vi "Controller Monitoring Loop.vi"(7 "Sync Objects":T1, 8 "error in (no error)":errorcluster, 11 "FOFB Configuration":T4={"FOFB Parameters"={"Network"={"FOFB Controller IP"="", "LNLS Control Network IP"="", "LNLS Control Network Power Supplies TCP Port"=0, "LNLS Control Network FOFB Configuration TCP Port"=0, "LNLS Control Network BPMs TCP Port"=0, "Data Server TCP Port"=0, "Monitoring Data TCP Port"=0, "Configuration GUI TCP Port"=0, "Storage Data TCP Port"=0, "Fast Command TCP Port"=0, "TCP Listening Timeout"=0, "Request Setpoints Rate"=0}, "Fast Acquisition"={"Acquisition Period"=0, "Data Buffer Size"=0, "Monitoring Period"=0}, "Response Matrix Measurement"={"Step Amplitude"=0.0, "Time Between Steps"=0, "Step Duration"=0, "Number of Averages"=0}, "Correction Algorithm"={"Correction Period"=0, "Reference Orbit Path"=path "", "Response Matrix Path"=path "", "Correction Matrix Path"=path "", "PID Horizontal Gain"=0.0, "PID Vertical Gain"=0.0, "PID Horizontal Integral Time"=0.0, "PID Vertical Integral Time"=0.0, "PID Horizontal Derivative Time"=0.0, "PID Vertical Derivative Time"=0.0, "Beam Current FOFB Threshold"=0.0, "Decouple H-V"=FALSE, "Use Additional BPM LPF"=FALSE, "BPM LPF Cutoff"=0.0}, "Acquisition Network"=[], "Actuation Network"=[]}, "Number of Acquisition Chassis"=0, "Number of Actuation Chassis"=0, "Number of BPM Readings"=0, "BPM Reading Names"=[], "Selected BPM Readings"=[0, 1, 2, 3, 4, 5, 6, 7, 8, 9, 10, 11, 12, 13, 14, 15, 16, 17, 18, 19, 20, 21, 22, 23, 24, 25, 26, 27, 28, 29, 30, 31, 32, 33, 34, 35, 36, 37, 38, 39, 40, 41, 42, 43, 44, 45, 46, 47, 48, 49], "Number of Correctors"=0, "Corrector Names"=[], "Selected Correctors"=[0, 1, 2, 3, 4, 5, 6, 7, 8, 9, 10, 11, 12, 13, 14, 15, 16, 17, 18, 19, 20, 21, 22, 23, 24, 25, 26, 27, 28, 29, 30, 31, 32, 33, 34, 35, 36, 37, 38, 39, 40, 41, 42, 43, 44, 45, 46, 47, 48, 49], "Reference Orbit"=[], "Response Matrix"=[], "Correction Matrix"=[], "Acquisition Chassis Names"=[], "Actuation Chassis Names"=[], "Acquisition Variables"=[], "Actuation Variables"=[], "PS Matrix Mapping"=[], "Inverse PS Matrix Mapping"=[], "BPM Matrix Mapping"=[], "Inverse BPM Matrix Mapping"=[], "Response Matrix Beam Energy (MeV)"=0.0, "PID Parameters"=[], "BPM Planes"=[], "Corrector Planes"=[], "RMM Step Factor"=[]}) -> (0 "error out":errorcluster)   [LabVIEW 2011, in "Controller VIs.lvlib"]
uses:
  Controller VIs.lvlib
  Types Definitions/Type FOFB Configuration.ctl
  Types Definitions/Type FOFB Parameters.ctl
  Types Definitions/Type Network Configuration.ctl
  Types Definitions/Type FA Configuration.ctl
  Types Definitions/Type Response Matrix Measurement Configuration.ctl
  Types Definitions/Type Correction Algorithm Configuration.ctl
  Types Definitions/Type Acquisition Network Configuration.ctl
  Types Definitions/Type Actuation Network Configuration.ctl
  Types Definitions/Type PID Parameters.ctl
  Types Definitions/Type Synchronization Objects.ctl
  Types Definitions/Type Blocking Synchronization Objects.ctl
  Types Definitions/Type Monitoring Data.ctl
  Types Definitions/Type Operation Mode State.ctl
  Types Definitions/Type Diagnostics Data.ctl
  Types Definitions/Type CPU Loads Array.ctl
  Types Definitions/Type CPU Loads.ctl
  Types Definitions/Type Non-blocking Synchronization Objects.ctl
  Types Definitions/Type FOFB Variables.ctl
  Types Definitions/Type Actuation State.ctl
  Types Definitions/Type TCP State.ctl
  <vilib>/Platform/TimedLoop/XDataNode/timing_clust.ctl
  <vilib>/Platform/TimedLoop/XDataNode/nitl_modes.ctl
  <vilib>/Platform/TimedLoop/XDataNode/wakeup.ctl
  Controller Global Variables/Controller Actuation State.vi
  Controller Global Variables/LNLS Control FOFB Configuration Out.vi
  Controller Global Variables/Monitoring Data.vi
  <vilib>/Platform/TimedLoop/XDataNode/XDataNode.xnode
  Filter VIs.lvlib
  Type Definitions.lvlib
  <vilib>/NI_Real-Time Target Support.lvlib
  Controller Global Variables.lvlib
  <vilib>/Platform/TimedLoop/XDataNode/XDNodeRunTimeDep.lvlib
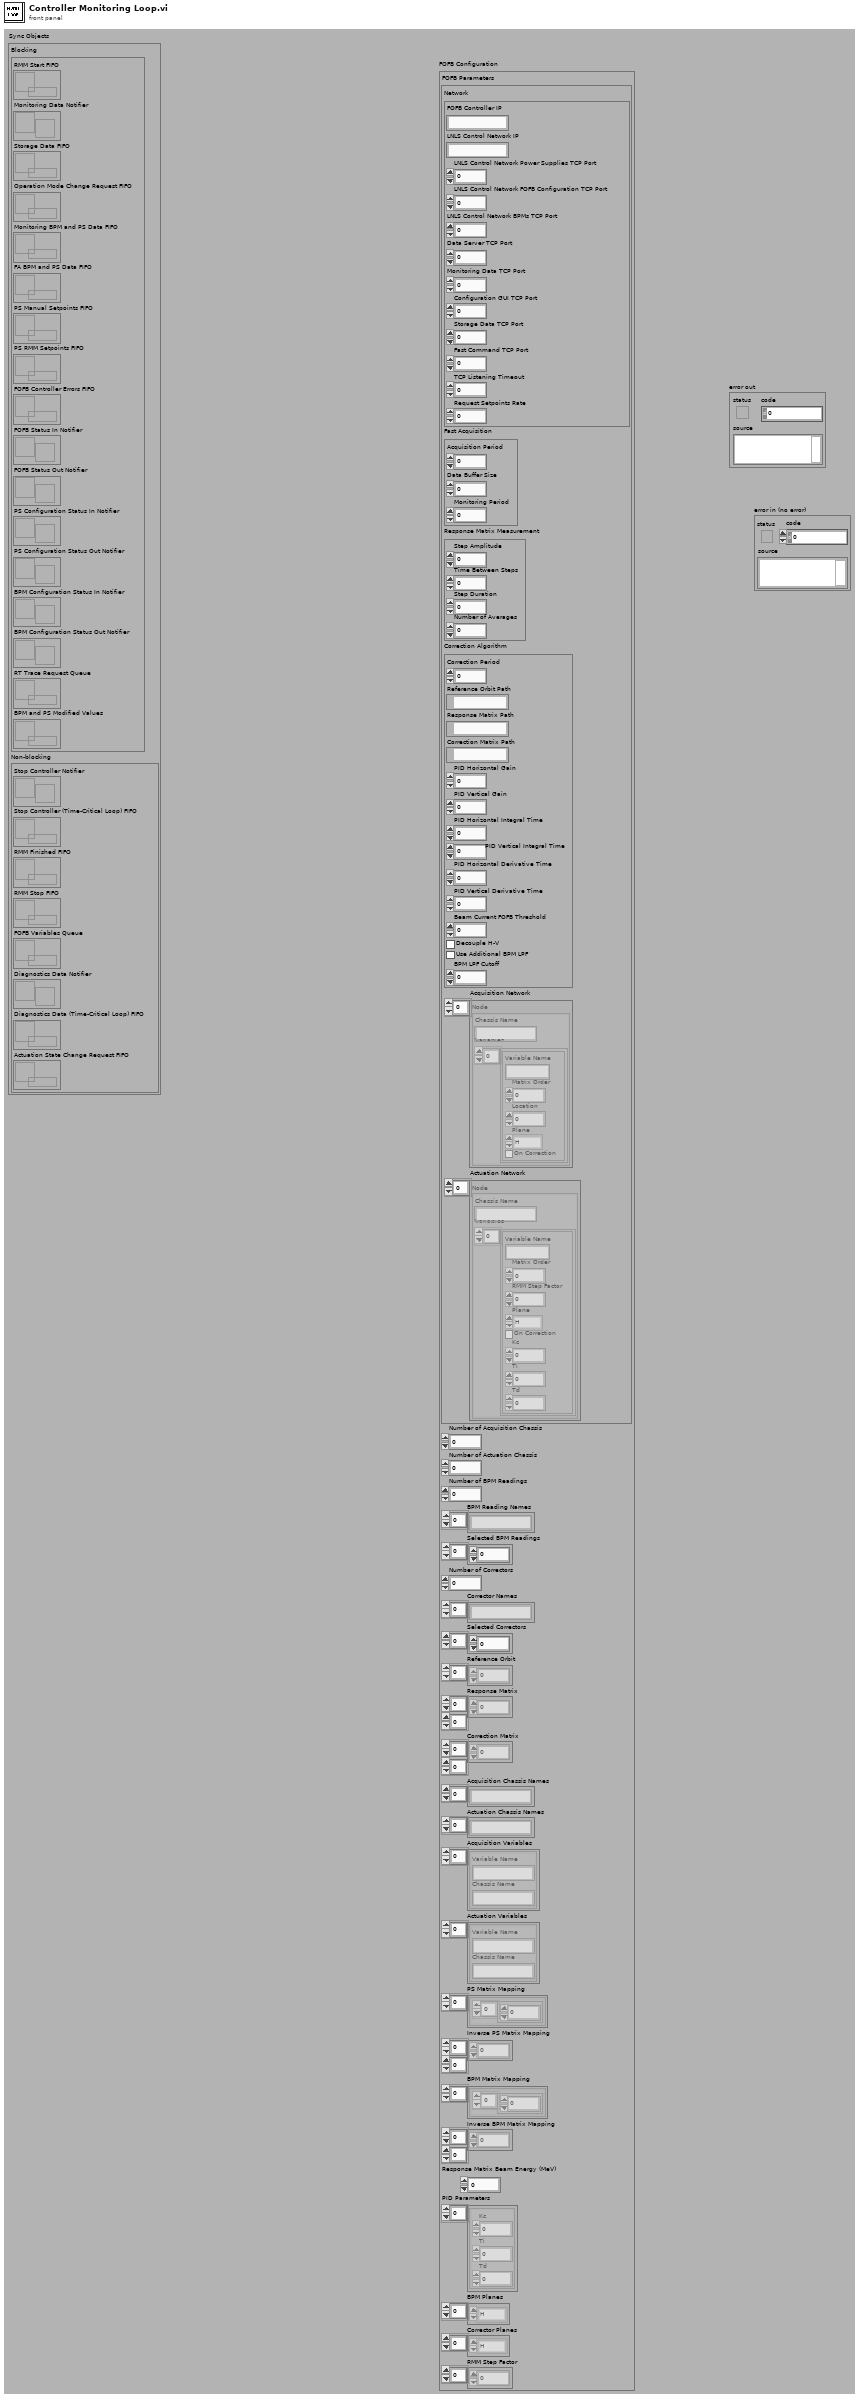
[diagram p1: front panel]
types:
  T1 = typedef "Type Definitions.lvlib/Type Synchronization Objects.ctl" = cluster{"Blocking":T2, "Non-blocking":T3}
  T2 = typedef "Type Definitions.lvlib/Type Blocking Synchronization Objects.ctl" = cluster{"RMM Start FIFO":refnum<k33>, "Monitoring Data Notifier":refnum<notifier>, "Storage Data FIFO":refnum<queue>, "Operation Mode Change Request FIFO":refnum<k33>, "Monitoring BPM and PS Data FIFO":refnum<k33>, "FA BPM and PS Data FIFO":refnum<k33>, "PS Manual Setpoints FIFO":refnum<k33>, "PS RMM Setpoints FIFO":refnum<k33>, "FOFB Controller Errors FIFO ":refnum<k33>, "FOFB Status In Notifier":refnum<notifier>, "FOFB Status Out Notifier":refnum<notifier>, "PS Configuration Status In Notifier":refnum<notifier>, "PS Configuration Status Out Notifier":refnum<notifier>, "BPM Configuration Status In Notifier":refnum<notifier>, "BPM Configuration Status Out Notifier":refnum<notifier>, "RT Trace Request Queue":refnum<queue>, "BPM and PS Modified Values":refnum<k33>}
  T3 = typedef "Type Definitions.lvlib/Type Non-blocking Synchronization Objects.ctl" = cluster{"Stop Controller Notifier":refnum<notifier>, "Stop Controller (Time-Critical Loop) FIFO":refnum<k33>, "RMM Finished FIFO":refnum<k33>, "RMM Stop FIFO":refnum<k33>, "FOFB Variables Queue":refnum<queue>, "Diagnostics Data Notifier":refnum<notifier>, "Diagnostics Data (Time-Critical Loop) FIFO":refnum<k33>, "Actuation State Change Request FIFO":refnum<k33>}
  T4 = typedef "Type Definitions.lvlib/Type FOFB Configuration.ctl" = cluster{"FOFB Parameters":T5, "Number of Acquisition Chassis":i32, "Number of Actuation Chassis":i32, "Number of BPM Readings":i32, "BPM Reading Names":string[], "Selected BPM Readings":u32[], "Number of Correctors":i32, "Corrector Names":string[], "Selected Correctors":u32[], "Reference Orbit":dbl[], "Response Matrix":dbl[][], "Correction Matrix":dbl[][], "Acquisition Chassis Names":string[], "Actuation Chassis Names":string[], "Acquisition Variables":cluster{"Variable Name":string, "Chassis Name":string}[], "Actuation Variables":cluster{"Variable Name":string, "Chassis Name":string}[], "PS Matrix Mapping":cluster{u32[]}[], "Inverse PS Matrix Mapping":u32[][], "BPM Matrix Mapping":cluster{u32[]}[], "Inverse BPM Matrix Mapping":u32[][], "Response Matrix Beam Energy (MeV)":dbl, "PID Parameters":T12[], "BPM Planes":enum8{"H", "V"}[], "Corrector Planes":enum8{"H", "V"}[], "RMM Step Factor":dbl[]}
  T5 = typedef "Type Definitions.lvlib/Type FOFB Parameters.ctl" = cluster{"Network":T6, "Fast Acquisition":T7, "Response Matrix Measurement":T8, "Correction Algorithm":T9, "Acquisition Network":T10, "Actuation Network":T11}
  T6 = typedef "Type Definitions.lvlib/Type Network Configuration.ctl" = cluster{"FOFB Controller IP":string, "LNLS Control Network IP":string, "LNLS Control Network Power Supplies TCP Port":u16, "LNLS Control Network FOFB Configuration TCP Port":u16, "LNLS Control Network BPMs TCP Port":u16, "Data Server TCP Port":u16, "Monitoring Data TCP Port":u16, "Configuration GUI TCP Port":u16, "Storage Data TCP Port":u16, "Fast Command TCP Port":u16, "TCP Listening Timeout":i32, "Request Setpoints Rate":u16}
  T7 = typedef "Type Definitions.lvlib/Type FA Configuration.ctl" = cluster{"Acquisition Period":u32, "Data Buffer Size":u32, "Monitoring Period":u32}
  T8 = typedef "Type Definitions.lvlib/Type Response Matrix Measurement Configuration.ctl" = cluster{"Step Amplitude":dbl, "Time Between Steps":u32, "Step Duration":u32, "Number of Averages":u32}
  T9 = typedef "Type Definitions.lvlib/Type Correction Algorithm Configuration.ctl" = cluster{"Correction Period":u32, "Reference Orbit Path":path, "Response Matrix Path":path, "Correction Matrix Path":path, "PID Horizontal Gain":dbl, "PID Vertical Gain":dbl, "PID Horizontal Integral Time":dbl, "PID Vertical Integral Time":dbl, "PID Horizontal Derivative Time":dbl, "PID Vertical Derivative Time":dbl, "Beam Current FOFB Threshold":dbl, "Decouple H-V":bool, "Use Additional BPM LPF":bool, "BPM LPF Cutoff":dbl}
  T10 = typedef "Type Definitions.lvlib/Type Acquisition Network Configuration.ctl" = cluster{"Chassis Name":string, "Variables":cluster{"Variable Name":string, "Matrix Order":u32, "Location":dbl, "Plane":enum8{"H", "V"}, "On Correction":bool}[]}[]
  T11 = typedef "Type Definitions.lvlib/Type Actuation Network Configuration.ctl" = cluster{"Chassis Name":string, "Variables":cluster{"Variable Name":string, "Matrix Order":u32, "RMM Step Factor":dbl, "Plane":enum8{"H", "V"}, "On Correction":bool, "Kc":dbl, "Ti":dbl, "Td":dbl}[]}[]
  T12 = typedef "Type Definitions.lvlib/Type PID Parameters.ctl" = cluster{"Kc":fxp<+/-,16,8>, "Ti":fxp<+/-,16,8>, "Td":fxp<+/-,16,8>}
  T13 = typedef "Type Definitions.lvlib/Type TCP State.ctl" = enum16{"Idle", "Wait Connection", "Read Data", "Process Data", "Write Data", "Close Connection"}
  T14 = typedef "XDNodeRunTimeDep.lvlib/timing_clust.ctl" = cluster{"Expected End [f-1]":u64, "Actual End [f-1]":u64, "Finished Late? [f-1]":bool, "Expected End [i-1]":u64, "Actual End [i-1]":u64, "Finished Late? [i-1]":bool, "Expected Start [i]":u64, "Actual Start [i]":u64, "Expected Start [f]":u64, "Actual Start [f]":u64, "Source Name":string, "Structure Name":string, "Period":i64, "Deadline":i64, "Offset":i64, "Start":i64, "Priority":i32, "Timeout":i32, "Mode":T15, "Wakeup Reason":T16, "Error":errorcluster, "Source Type":string, "Secondary Source Type":string, "Global End Time":u64, "Global Start Time":u64, "Frame Duration":u64, "Iteration Duration":u64, "Assigned CPU":i32, "I/O Scan Engine Mode":u32}
  T15 = typedef "XDNodeRunTimeDep.lvlib/nitl_modes.ctl" = enum32{"No Change", "Process missed periods, maintain original phase", "Discard missed periods, maintain original phase", "Process missed periods, ignore original phase", "Discard missed periods, ignore original phase"}
  T16 = typedef "XDNodeRunTimeDep.lvlib/wakeup.ctl" = enum32{"Normal", "Aborted", "Asynchronous wakeup", "Timing source error", "Timed loop error", "Timeout"}
  T17 = typedef "Type Definitions.lvlib/Type Monitoring Data.ctl" = cluster{"Timestamp":timestamp, "BPM Readings":dbl[], "PS Readings":dbl[], "PS FOFB Setpoints":dbl[], "PS Status per Rack":u8[], "PS ON-OFF per Rack":u8[], "Operation Mode":T18, "Diagnostics Data":T19, "Controller Status Table":i32[]}
  T18 = typedef "Type Definitions.lvlib/Type Operation Mode State.ctl" = enum8{"Idle Mode", "Manual Mode", "FOFB Mode", "RMM Mode"}
  T19 = typedef "Type Definitions.lvlib/Type Diagnostics Data.ctl" = cluster{"Time-Critical Loop Missed Iterations":u32, "Time-Critical Loop Execution Time (usec)":u32, "Available Memory (bytes)":u32, "CPU Loads Array":T20}
  T20 = typedef "Type Definitions.lvlib/Type CPU Loads Array.ctl" = T21[]
  T21 = typedef "Type Definitions.lvlib/Type CPU Loads.ctl" = cluster{"Total (%)":dbl, "Time Critical (%)":dbl, "Timed Structures (%)":dbl, "High (%)":dbl, "Above Normal (%)":dbl, "Normal (%)":dbl, "Background (%)":dbl, "Idle (%)":dbl, "ISR (%)":dbl}
  T22 = typedef "Type Definitions.lvlib/Type Actuation State.ctl" = enum8{"Only reading", "Manual", "FOFB Initialization", "FOFB", "FOFB Stopping", "RMM Initialization", "RMM", "RMM Stopping"}
  T23 = typedef "Type Definitions.lvlib/Type Control FOFB Configuration Out.ctl" = cluster{"Status":u16, "Operation Mode":T18, "PID Horizontal Gain":sgl, "PID Vertical Gain":sgl, "PID Horizontal Integral Time":sgl, "PID Vertical Integral Time":sgl, "PID Horizontal Derivative Time":sgl, "PID Vertical Derivative Time":sgl, "Fast Command Enabled":bool, "RMS Horizontal Distortion":dbl, "RMS Vertical Distortion":dbl, "Timestamp":dbl}
  T24 = typedef "NI_Real-Time Target Support.lvlib/RT CPU Load.ctl" = cluster{"Total (%)":dbl, "Time Critical (%)":dbl, "Timed Structures (%)":dbl, "High (%)":dbl, "Above Normal (%)":dbl, "Normal (%)":dbl, "Background (%)":dbl, "Idle (%)":dbl, "ISR (%)":dbl}
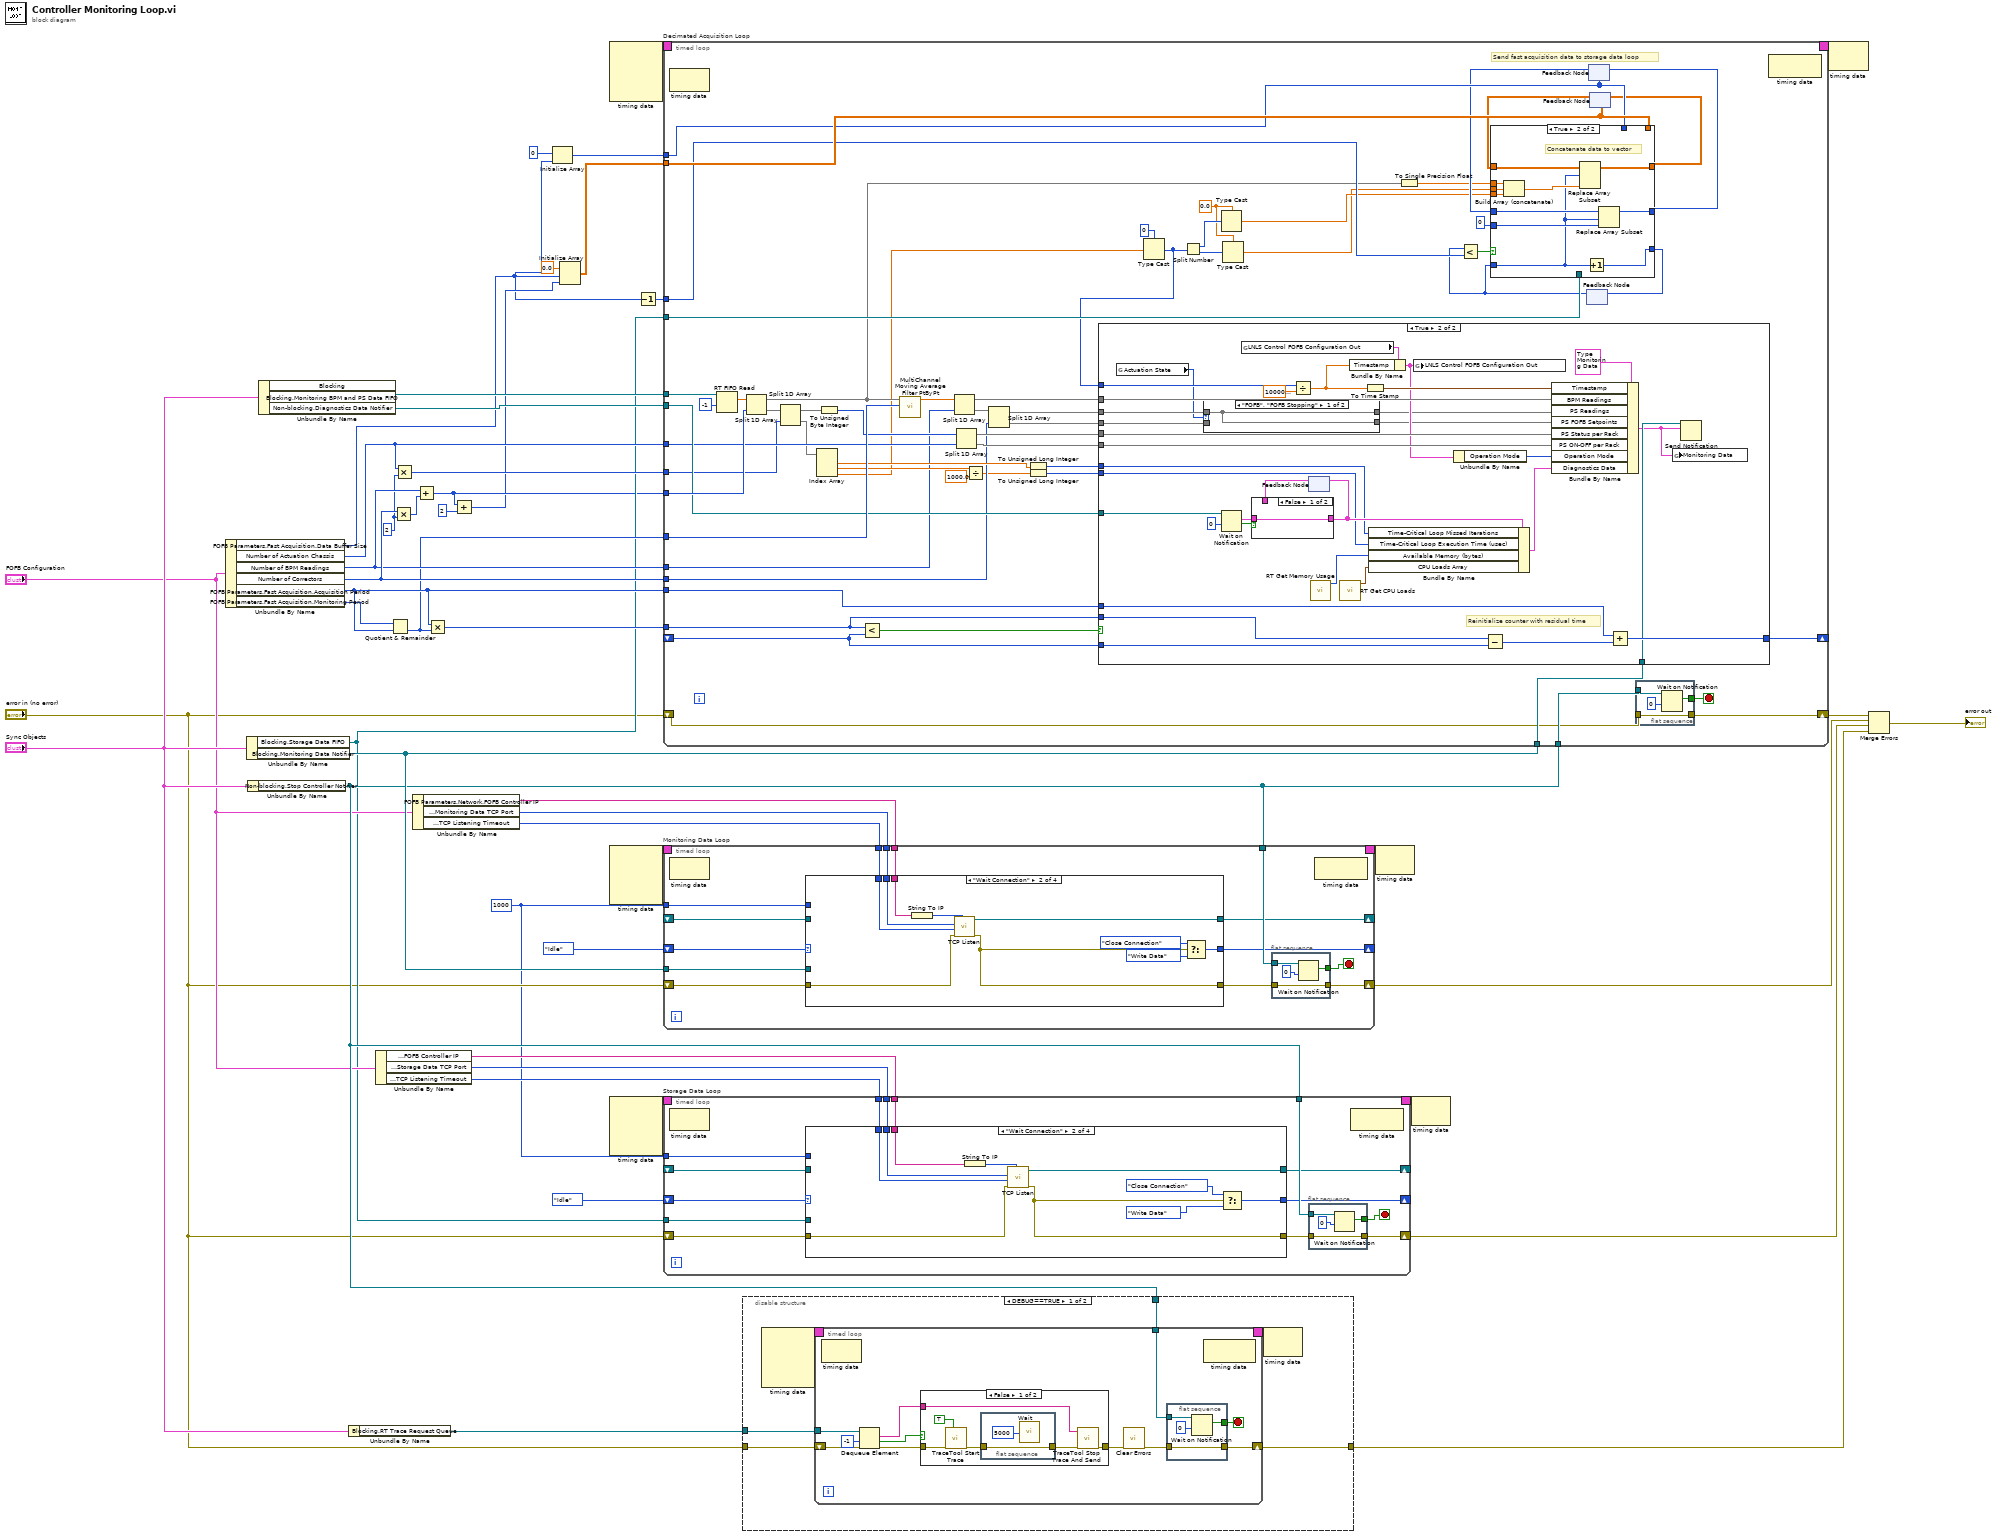
[diagram p0: block diagram]
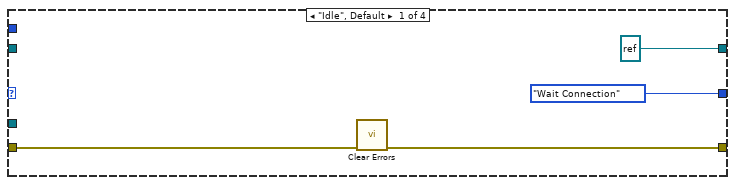
[diagram p2: hidden frame]
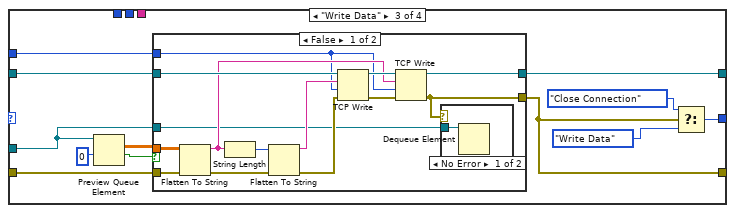
[diagram p3: hidden frame]
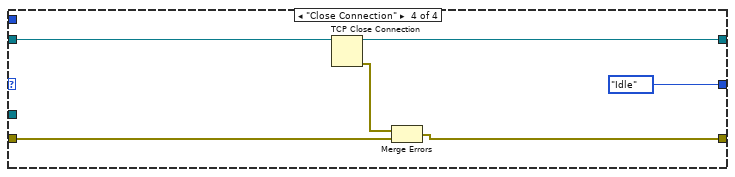
[diagram p6: hidden frame]
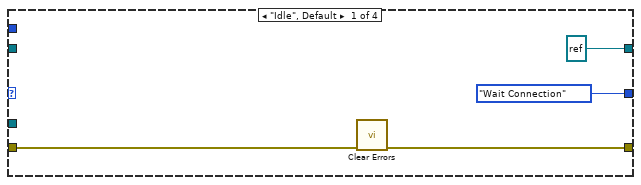
[diagram p7: hidden frame]
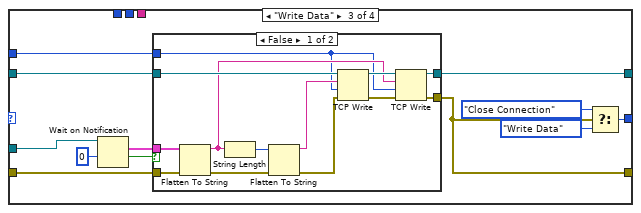
[diagram p8: hidden frame]
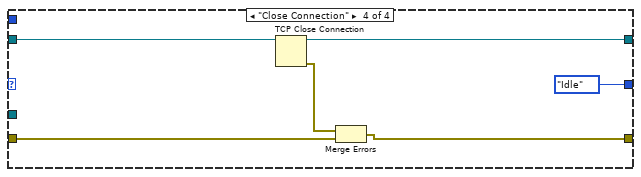
[diagram p10: hidden frame]
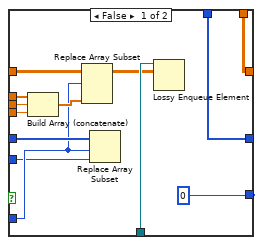
[diagram p13: hidden frame]
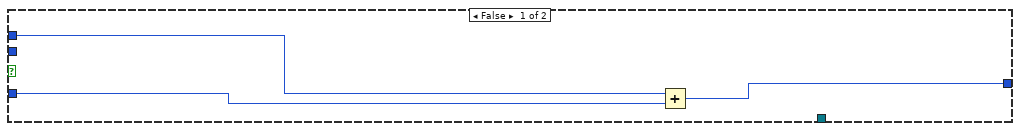
[diagram p14: hidden frame]
diagram:
  w1 = 1000 ("TCP Listening Timeout")
  w37 = 2 ("y")
  n1 = Unbundle By Name("FOFB Configuration") -> ("FOFB Parameters.Fast Acquisition.Data Buffer Size"=w2:u32, "Number of Actuation Chassis"=w36:i32, "Number of BPM Readings"=w40:i32, "Number of Correctors"=w41:i32, "FOFB Parameters.Fast Acquisition.Acquisition Period"=w34:u32, "FOFB Parameters.Fast Acquisition.Monitoring Period"=w24:u32)
  n2 = Unbundle By Name("Sync Objects") -> ("Blocking.Storage Data FIFO"=w12:refnum<queue>, "Blocking.Monitoring Data Notifier"=w26:refnum<notifier>)
  n3 = Unbundle By Name("Sync Objects") -> ("Non-blocking.Stop Controller Notifier"=w23:refnum<notifier>)
  n4 = Unbundle By Name("Sync Objects") -> ("Blocking.Monitoring BPM and PS Data FIFO"=w13:refnum<k33>, "Non-blocking.Diagnostics Data Notifier"=w38:refnum<notifier>)  [unwired: 1 out]
  n5 = Unbundle By Name("Sync Objects") -> ("Blocking.RT Trace Request Queue"=w30:refnum<queue>)
  n6 = Unbundle By Name("FOFB Configuration") -> ("FOFB Parameters.Network.FOFB Controller IP"=w21:string, "FOFB Parameters.Network.Storage Data TCP Port"=w20:u16, "FOFB Parameters.Network.TCP Listening Timeout"=w19:i32)
  n7 = Quotient & Remainder(x=w24, y=w34) -> (floor(x/y)=w33:u32)  [unwired: 1 out]
  n8 = Multiply(x=w41, y=w37) -> (x*y=w39:i32)
  n9 = Multiply(x=w36, y=w37) -> (x*y=w35:i32)
  n10 = Unbundle By Name("FOFB Configuration") -> ("FOFB Parameters.Network.FOFB Controller IP"=w48:string, "FOFB Parameters.Network.Monitoring Data TCP Port"=w43:u16, "FOFB Parameters.Network.TCP Listening Timeout"=w47:i32)
  n11 = Add(x=w40, y=w39) -> (x+y=w5:i32)
  n12 = Multiply(x=w34, y=w33) -> (x*y=w25:u32)
  n13 = Add(x=w5, y=2) -> (x+y=w4:i32)
  n14 = Initialize Array(u64 0 ("Timestamp"), w2) -> (w14:u64[])
  n15 = Initialize Array(sgl 0.0 ("element"), w2, w4) -> (w7:sgl[][])
  n16 = node-c288() -> (w32:T14)  [unwired: 4 in]
  n17 = node-c288() -> (w28:T14)  [unwired: 4 in]
  n18 = node-c288() -> (w10:T14)  [unwired: 4 in]
  n19 = Decrement(x=w2) -> (x-1=w3:u32)
  n20 = timed-loop "Decimated Acquisition Loop" {
    shift-right: [w78] -> w46
    shift-left: "error in (no error)" -> [w79]
    tunnel: w23 -> [w106]
    tunnel: w40 -> [w76]
    tunnel: w41 -> [w75]
    tunnel: w34 -> [w101]
    tunnel: w25 -> [w100]
    tunnel: w26 -> [w98]
    tunnel: w33 -> [w97]
    shift-right: [w95] -> _
    shift-left: _ -> [w96]
    tunnel: w5 -> [w92]
    tunnel: w38 -> [w91]
    tunnel: w36 -> [w87]
    tunnel: w35 -> [w84]
    timing: w32 -> [_]
    timing-out: [_] -> w31
    tunnel: w7 -> [w72]
    tunnel: w3 -> [w60]
    tunnel: w14 -> [w71]
    tunnel: w13 -> [w70]
    tunnel: w12 -> [w69]
    stop <- w107 stop-if-true
    w54 = sgl 0.0 ("single precision float")
    # "Send fast acquisition data to storage data loop"
    n21 = node-c288() -> ()  [unwired: 1 in, 1 out]
    n22 = RT FIFO Read(0:w70, 2:-1 ("timeout in ms (0)")) -> (9:w93:dbl[])  [unwired: 2 in, 4 out]
    n23 = Split 1D Array(array=w93, index=w92) -> (first subarray=w58:dbl[], second subarray=w86:dbl[])
    n24 = Split 1D Array(array=w86, index=w84) -> (first subarray=w85:dbl[], second subarray=w61:dbl[])
    n25 = Index Array(array=w61) -> (element #1=w82:dbl, element #2=w81:dbl, element #3=w51:dbl)  [unwired: 3 in]
    n26 = To Unsigned Byte Integer(number=w85) -> (unsigned 8bit integer=w90:u8[])
    n27 = Less?(x=w100, y=w96) -> (x < y?=w99:bool)
    n28 = call "MultiChannel Moving Average Filter PtByPt.vi"("Number of Averages"=w97, "X"=w58) -> ("Filtered X"=w105:dbl[])  [unwired: 9 in]
    n29 = Split 1D Array(array=w105, index=w76) -> (first subarray=w77:dbl[], second subarray=w104:dbl[])
    n30 = Split 1D Array(array=w90, index=w87) -> (first subarray=w89:u8[], second subarray=w88:u8[])
    n31 = Divide(x=w81, y=1000.0) -> (x/y=w74:dbl)
    n32 = Split 1D Array(array=w104, index=w75) -> (first subarray=w103:dbl[], second subarray=w102:dbl[])
    n33 = To Unsigned Long Integer(number=w82) -> (unsigned 32bit integer=w83:u32)
    n34 = To Unsigned Long Integer(number=w74) -> (unsigned 32bit integer=w73:u32)
    n35 = Type Cast(type=u64 0 ("n"), x=w51) -> (*(type *) &x=w49:u64)
    n36 = case shown="True" w99 {
      tunnel: w77 -> [_ w169]
      tunnel: w103 -> [_ w144]
      tunnel: w102 -> [_ w145]
      tunnel: [w138 w173] -> w95
      tunnel: w96 -> [w139 w172]
      tunnel: w100 -> [_ w171]
      tunnel: w101 -> [w140 w170]
      tunnel: w98 -> [_ w153]
      tunnel: w89 -> [_ w165]
      tunnel: w91 -> [_ w159]
      tunnel: w88 -> [_ w158]
      tunnel: w83 -> [_ w155]
      tunnel: w73 -> [_ w156]
      tunnel: w49 -> [_ w150]
      frame False {
        n37 = Add(x=w140, y=w139) -> (x+y=w138:u32)
      }
      frame True {
        # "Reinitialize counter with residual time"
        n38 = global read "Controller Actuation State.vi" "Actuation State"() -> (w143:T22)
        n39 = case shown="\"FOFB\", \"FOFB Stopping\"" w143 {
          tunnel: w145 -> [_ w176]
          tunnel: w144 -> [w175 w177]
          tunnel: [w175 w177] -> w142
          tunnel: [w175 w176] -> w141
          frame "FOFB", "FOFB Stopping" {
          }
          frame "Manual", Default {
          }
        }
        n40 = Wait on Notification(notifier=w159, timeout in ms (-1)=0) -> (notification=w161:T19, timed out?=w162:bool)  [unwired: 2 in, 2 out]
        n41 = global read "LNLS Control FOFB Configuration Out.vi" "LNLS Control FOFB Configuration Out"() -> (w149:T23)
        n42 = Divide(x=w150, y=1000000000.0) -> (x/y=w147:dbl)
        n43 = feedback #1() -> (w163:T19)  [unwired: 1 in]
        n44 = case shown="False" w162 {
          tunnel: [w178 w179] -> w160
          tunnel: w161 -> [w178 _]
          tunnel: w163 -> [_ w179]
          frame False {
          }
          frame True {
          }
        }
        n45 = feedback-in #1(w160) -> ()
        n46 = call <vilib>:"RT Get Memory Usage.vi"() -> ("total (bytes)"=w157:u32)  [unwired: 8 in, 3 out]
        n47 = call <vilib>:"RT Get CPU Loads.vi"() -> ("CPU loads"=w167:T24[])  [unwired: 10 in, 1 out]
        n48 = Bundle By Name(cluster=w149, "Timestamp"=w147) -> (w146:T23)
        n49 = To Time Stamp(1:w147) -> (0:w148:timestamp)
        n50 = Bundle By Name(cluster=w160, "Time-Critical Loop Missed Iterations"=w155, "Time-Critical Loop Execution Time (usec)"=w156, "Available Memory (bytes)"=w157, "CPU Loads Array"=w167) -> (w166:T19)
        n51 = global write "LNLS Control FOFB Configuration Out.vi" "LNLS Control FOFB Configuration Out"(w146) -> ()
        n52 = Unbundle By Name(w146) -> ("Operation Mode"=w154:T18)
        n53 = Subtract(x=w171, y=w172) -> (x-y=w174:u32)
        n54 = Bundle By Name(cluster=T17 {"Timestamp"=timestamp(0 s since 1904-01-01), "BPM Readings"=[], "PS Readings"=[], "PS FOFB Setpoints"=[], "PS Status per Rack"=[], "PS ON-OFF per Rack"=[], "Operation Mode"=enum."Idle Mode", "Diagnostics Data"={"Time-Critical Loop Missed Iterations"=0, "Time-Critical Loop Execution Time (usec)"=0, "Available Memory (bytes)"=0, "CPU Loads Array"=[]}, "Controller Status Table"=[]} ("output cluster"), "Timestamp"=w148, "BPM Readings"=w169, "PS Readings"=w142, "PS FOFB Setpoints"=w141, "PS Status per Rack"=w165, "PS ON-OFF per Rack"=w158, "Operation Mode"=w154, "Diagnostics Data"=w166) -> (w152:T17)
        n55 = Add(x=w170, y=w174) -> (x+y=w173:u32)
        n56 = global write "Monitoring Data.vi" "Monitoring Data"(w152) -> ()
        n57 = Send Notification(notification=w152, notifier=w153) -> ()  [unwired: 1 in, 2 out]
      }
    }
    n58 = Split Number(x=w49) -> (hi(x)=w55:u32, lo(x)=w56:u32)
    n59 = Type Cast(type=w54, x=w55) -> (*(type *) &x=w53:sgl)
    n60 = Type Cast(type=w54, x=w56) -> (*(type *) &x=w52:sgl)
    n61 = To Single Precision Float(number=w58) -> (single precision float=w57:sgl[])
    n62 = feedback #2() -> (w59:i32)  [unwired: 1 in]
    n63 = Less?(x=w59, y=w60) -> (x < y?=w63:bool)
    n64 = feedback #3(w71) -> (w66:u64[])
    n65 = feedback #4(w72) -> (w67:sgl[][])
    n66 = case shown="True" w63 {
      tunnel: [0 ("x+1") w129] -> w64
      tunnel: [w118 w128] -> w68
      tunnel: w67 -> [w120 w131]
      tunnel: w66 -> [w115 w127]
      tunnel: u64 0 ("element") -> [w113 w126]
      tunnel: [w116 w125] -> w65
      tunnel: w59 -> [w114 w124]
      tunnel: w72 -> [w118 _]
      tunnel: w71 -> [w116 _]
      tunnel: w69 -> [w112 _]
      tunnel: w52 -> [w109 w121]
      tunnel: w57 -> [w110 w123]
      tunnel: w53 -> [w108 w122]
      frame False {
        n67 = Build Array (concatenate)(w110, w109, w108) -> (w119:sgl[])
        n68 = Replace Array Subset(array=w120, new element=w119, index (row)=w114) -> (w111:sgl[][])  [unwired: 1 in]
        n69 = Replace Array Subset(array=w115, new element=w113, index=w114) -> ()  [unwired: 1 out]
        n70 = Lossy Enqueue Element(queue=w112, element=w111) -> ()  [unwired: 1 in, 4 out]
      }
      frame True {
        # "Concatenate data to vector"
        n71 = Build Array (concatenate)(w123, w121, w122) -> (w130:sgl[])
        n72 = Replace Array Subset(array=w131, new element=w130, index (row)=w124) -> (w128:sgl[][])  [unwired: 1 in]
        n73 = Increment(x=w124) -> (x+1=w129:i32)
        n74 = Replace Array Subset(array=w127, new element=w126, index=w124) -> (w125:u64[])
      }
    }
    n75 = feedback-in #2(w64) -> ()
    n76 = feedback-in #3(w65) -> ()
    n77 = feedback-in #4(w68) -> ()
    n78 = flat-sequence {
      tunnel: [w135] -> w107
      tunnel: w106 -> [w134]
      tunnel: w79 -> [w133]
      tunnel: [w133] -> w78
      frame #0 {
        n79 = Wait on Notification(notifier=w134, timeout in ms (-1)=0) -> (notification=w135:bool)  [unwired: 2 in, 3 out]
      }
    }
    n80 = node-c288() -> ()  [unwired: 1 in, 1 out]
  }
  n81 = timed-loop "Monitoring Data Loop" {
    tunnel: w48 -> [w193]
    tunnel: w43 -> [w192]
    tunnel: w47 -> [w191]
    shift-right: [w184] -> w45
    shift-left: "error in (no error)" -> [w182]
    tunnel: w23 -> [w189]
    tunnel: w26 -> [w181]
    shift-right: [w187] -> _
    shift-left: Type_TCP_State."Idle" ("f") -> [w188]
    shift-right: [w185] -> _
    shift-left: _ -> [w186]
    timing: w28 -> [_]
    timing-out: [_] -> w27
    tunnel: w1 -> [w180]
    stop <- w190 stop-if-true
    n82 = node-c288() -> ()  [unwired: 1 in, 1 out]
    n83 = case shown="\"Wait Connection\"" w188 {
      tunnel: [refnum<k5> refnum ("connection ID") w213 w225 w246] -> w185
      tunnel: [Type_TCP_State."Wait Connection" ("f") w212 w224 Type_TCP_State."Idle" ("f")] -> w187
      tunnel: [w200 w208 w220 w241] -> w183
      tunnel: w182 -> [w201 w209 w216 w242]
      tunnel: w186 -> [_ _ w221 w244]
      tunnel: w193 -> [_ w205 _ _]
      tunnel: w192 -> [_ w207 _ _]
      tunnel: w191 -> [_ w204 _ _]
      tunnel: w181 -> [_ _ w219 _]
      tunnel: w180 -> [_ _ w214 _]
      frame "Idle", Default {
        n84 = call <vilib>:"Clear Errors.vi"("error in (no error)"=w201) -> ("error out"=w200:errorcluster)  [unwired: 6 in]
      }
      frame "Wait Connection" {
        n85 = String To IP(1:w205) -> (0:w206:u32)
        n86 = call <vilib>:"TCP Listen.vi"("net address"=w206, "error in (no error)"=w209, "timeout ms (wait forever: -1)"=w204, "port"=w207) -> ("error out"=w208:errorcluster, "connection ID"=w213:refnum<k5>)  [unwired: 3 in, 3 out]
        n87 = Select(t=Type_TCP_State."Close Connection" ("f"), s=w208, f=Type_TCP_State."Write Data") -> (s? t:f=w212:T13)
      }
      frame "Write Data" {
        n88 = Wait on Notification(notifier=w219, timeout in ms (-1)=0) -> (notification=w218:T17, timed out?=w215:bool)  [unwired: 2 in, 2 out]
        n89 = case shown="False" w215 {
          tunnel: [w238 w240] -> w225
          tunnel: w221 -> [w236 w240]
          tunnel: w214 -> [w229 _]
          tunnel: [w228 w239] -> w220
          tunnel: w218 -> [w227 _]
          tunnel: w216 -> [w226 w239]
          frame False {
            n90 = Flatten To String(anything=w227, error in (no error)=w226) -> (data string=w232:string, error out=w231:errorcluster)  [unwired: 2 in, 1 out]
            n91 = String Length(string=w232) -> (length=w234:i32)
            n92 = Flatten To String(anything=w234, error in (no error)=w231) -> (data string=w233:string, error out=w230:errorcluster)  [unwired: 2 in, 1 out]
            n93 = TCP Write(connection ID=w236, data in=w233, error in (no error)=w230, 9:w229) -> (connection ID out=w237:refnum<k5>, error out=w235:errorcluster)  [unwired: 1 out]
            n94 = TCP Write(connection ID=w237, data in=w232, error in (no error)=w235, 9:w229) -> (connection ID out=w238:refnum<k5>, error out=w228:errorcluster)  [unwired: 1 out]
          }
          frame True {
          }
        }
        n95 = Select(t=Type_TCP_State."Close Connection" ("f"), s=w220, f=Type_TCP_State."Write Data") -> (s? t:f=w224:T13)
      }
      frame "Close Connection" {
        n96 = TCP Close Connection(connection ID=w244) -> (connection ID out=w246:refnum<k5>, error out=w243:errorcluster)  [unwired: 2 in]
        n97 = Merge Errors(w243, w242) -> (w241:errorcluster)
      }
    }
    n98 = flat-sequence {
      tunnel: [w198] -> w190
      tunnel: w189 -> [w197]
      tunnel: [w196] -> w184
      tunnel: w183 -> [w196]
      frame #0 {
        n99 = Wait on Notification(notifier=w197, timeout in ms (-1)=0) -> (notification=w198:bool)  [unwired: 2 in, 3 out]
      }
    }
    n100 = node-c288() -> ()  [unwired: 1 in, 1 out]
  }
  n101 = timed-loop "Storage Data Loop" {
    tunnel: w21 -> [w260]
    tunnel: w20 -> [w259]
    tunnel: w19 -> [w258]
    shift-right: [w251] -> w17
    shift-left: "error in (no error)" -> [w249]
    tunnel: w23 -> [w256]
    tunnel: w12 -> [w248]
    shift-right: [w254] -> _
    shift-left: Type_TCP_State."Idle" ("f") -> [w255]
    shift-right: [w252] -> _
    shift-left: _ -> [w253]
    timing: w10 -> [_]
    timing-out: [_] -> w9
    tunnel: w1 -> [w247]
    stop <- w257 stop-if-true
    n102 = node-c288() -> ()  [unwired: 1 in, 1 out]
    n103 = case shown="\"Wait Connection\"" w255 {
      tunnel: [refnum<k5> refnum ("connection ID") w280 w292 w315] -> w252
      tunnel: [Type_TCP_State."Wait Connection" ("f") w279 w291 Type_TCP_State."Idle" ("f")] -> w254
      tunnel: [w267 w275 w287 w310] -> w250
      tunnel: w249 -> [w268 w276 w286 w311]
      tunnel: w253 -> [_ _ w288 w313]
      tunnel: w260 -> [_ w272 _ _]
      tunnel: w259 -> [_ w274 _ _]
      tunnel: w258 -> [_ w271 _ _]
      tunnel: w248 -> [_ _ w284 _]
      tunnel: w247 -> [_ _ w281 _]
      frame "Idle", Default {
        n104 = call <vilib>:"Clear Errors.vi"("error in (no error)"=w268) -> ("error out"=w267:errorcluster)  [unwired: 6 in]
      }
      frame "Wait Connection" {
        n105 = String To IP(1:w272) -> (0:w273:u32)
        n106 = call <vilib>:"TCP Listen.vi"("net address"=w273, "error in (no error)"=w276, "timeout ms (wait forever: -1)"=w271, "port"=w274) -> ("error out"=w275:errorcluster, "connection ID"=w280:refnum<k5>)  [unwired: 3 in, 3 out]
        n107 = Select(t=Type_TCP_State."Close Connection" ("f"), s=w275, f=Type_TCP_State."Write Data") -> (s? t:f=w279:T13)
      }
      frame "Write Data" {
        n108 = Preview Queue Element(queue=w284, timeout in ms (-1)=0) -> (element=w283:sgl[][], timed out?=w285:bool)  [unwired: 1 in, 2 out]
        n109 = case shown="False" w285 {
          tunnel: [w306 w309] -> w292
          tunnel: w288 -> [w304 w309]
          tunnel: w281 -> [w297 _]
          tunnel: [w294 w308] -> w287
          tunnel: w283 -> [w296 _]
          tunnel: w286 -> [w295 w308]
          tunnel: w284 -> [w293 _]
          frame False {
            n110 = Flatten To String(anything=w296, error in (no error)=w295) -> (data string=w300:string, error out=w299:errorcluster)  [unwired: 2 in, 1 out]
            n111 = String Length(string=w300) -> (length=w302:i32)
            n112 = Flatten To String(anything=w302, error in (no error)=w299) -> (data string=w301:string, error out=w298:errorcluster)  [unwired: 2 in, 1 out]
            n113 = TCP Write(connection ID=w304, data in=w301, error in (no error)=w298, 9:w297) -> (connection ID out=w305:refnum<k5>, error out=w303:errorcluster)  [unwired: 1 out]
            n114 = TCP Write(connection ID=w305, data in=w300, error in (no error)=w303, 9:w297) -> (connection ID out=w306:refnum<k5>, error out=w294:errorcluster)  [unwired: 1 out]
            n115 = case shown="No Error" w294 {
              tunnel: w293 -> [w307 _]
              frame No Error {
                n116 = Dequeue Element(queue=w307) -> ()  [unwired: 2 in, 4 out]
              }
              frame Error {
              }
            }
          }
          frame True {
          }
        }
        n117 = Select(t=Type_TCP_State."Close Connection" ("f"), s=w287, f=Type_TCP_State."Write Data") -> (s? t:f=w291:T13)
      }
      frame "Close Connection" {
        n118 = TCP Close Connection(connection ID=w313) -> (connection ID out=w315:refnum<k5>, error out=w312:errorcluster)  [unwired: 2 in]
        n119 = Merge Errors(w312, w311) -> (w310:errorcluster)
      }
    }
    n120 = flat-sequence {
      tunnel: [w265] -> w257
      tunnel: w256 -> [w264]
      tunnel: [w263] -> w251
      tunnel: w250 -> [w263]
      frame #0 {
        n121 = Wait on Notification(notifier=w264, timeout in ms (-1)=0) -> (notification=w265:bool)  [unwired: 2 in, 3 out]
      }
    }
    n122 = node-c288() -> ()  [unwired: 1 in, 1 out]
  }
  n123 = disable-structure shown="DEBUG==TRUE" {
    disable-tunnel: "error in (no error)" -> [w319 _]
    disable-tunnel: w30 -> [w318 _]
    disable-tunnel: w23 -> [w317 _]
    disable-tunnel: [w316 _] -> w18
    frame condition #0 (active) {
      n124 = node-c288() -> (w321:T14)  [unwired: 4 in]
      n125 = timed-loop {
        timing: w321 -> [_]
        timing-out: [_] -> w320
        tunnel: w318 -> [w330]
        shift-right: [w329] -> w316
        shift-left: w319 -> [w326]
        tunnel: w317 -> [w324]
        stop <- w327 stop-if-true
        n126 = node-c288() -> ()  [unwired: 1 in, 1 out]
        n127 = Dequeue Element(queue=w330, timeout in ms (-1)=-1, error in (no error)=w326) -> (element=w328:string, timed out?=w331:bool, error out=w325:errorcluster)  [unwired: 1 out]
        n128 = case shown="False" w331 {
          tunnel: [w341 w345] -> w323
          tunnel: w328 -> [w340 _]
          tunnel: w325 -> [w339 w345]
          frame False {
            n129 = call <vilib>:"TraceTool Start Trace.vi"("Detailed Tracing? (F)"=TRUE, "error in (no error)"=w339) -> ("error out"=w342:errorcluster)  [unwired: 8 in, 1 out]
            n130 = flat-sequence {
              tunnel: w342 -> [w343]
              tunnel: [w343] -> w337
              frame #0 {
                n131 = call "Wait"("Count(mSec)"=u32 5000) -> ()  [unwired: 1 out]
              }
            }
            n132 = call <vilib>:"TraceTool Stop Trace And Send.vi"("error in (no error)"=w337, "Trace Host Network Address"=w340) -> ("error out"=w341:errorcluster)  [unwired: 9 in]
          }
          frame True {
          }
        }
        n133 = call <vilib>:"Clear Errors.vi"("error in (no error)"=w323) -> ("error out"=w322:errorcluster)  [unwired: 6 in]
        n134 = flat-sequence {
          tunnel: [w335] -> w327
          tunnel: [w333] -> w329
          tunnel: w324 -> [w334]
          tunnel: w322 -> [w333]
          frame #0 {
            n135 = Wait on Notification(notifier=w334, timeout in ms (-1)=0) -> (notification=w335:bool)  [unwired: 2 in, 3 out]
          }
        }
        n136 = node-c288() -> ()  [unwired: 1 in, 1 out]
      }
      n137 = node-c288(w320) -> ()  [unwired: 1 out]
    }
    frame condition #1 {
    }
  }
  n138 = node-c288(w27) -> ()  [unwired: 1 out]
  n139 = node-c288(w9) -> ()  [unwired: 1 out]
  n140 = node-c288(w31) -> ()  [unwired: 1 out]
  n141 = Merge Errors(w46, w45, w17, w18) -> (→"error out":errorcluster)
